vi "AprilTagFieldLayout_New.vi"(9 "FieldWidth_Meters":dbl, 10 "FieldLength_Meters":dbl, 11 "AprilTags":T1[](array[typedef]) {"POSE3D"."Translation3d"."Z" format="%14.3f"; "POSE3D"."Translation3d"."Y" format="%14.3f"; "POSE3D"."Translation3d"."X" format="%14.3f"}) -> (3 "AprilTagFieldLayout":T6={"AprilTagMap"={}, "FieldLength"=0.0, "FieldWidth"=0.0, "OriginPosition "=enum."kBlueAllianceWallRightSide,", "OriginPose3d"={"Translation3d"={"X"=0.0, "Y"=0.0, "Z"=0.0}, "Rotation3d"={"Q_quaternion"={"R"=1.0, "V"=[0.0, 0.0, 0.0]}}}} {"OriginPose3d"."Translation3d"."Z" format="%14.3f"; "OriginPose3d"."Translation3d"."Y" format="%14.3f"; "OriginPose3d"."Translation3d"."X" format="%14.3f"})   [LabVIEW 2019, in "Trajectory_Library.lvlib"]
uses:
  TypeDef/AprilTag.ctl
  TypeDef/POSE3D.ctl
  TypeDef/TRANSLATION3D.ctl
  TypeDef/ROTATION3D.ctl
  TypeDef/QUATERNION.ctl
  Trajectory_Library.lvlib
  Enum/AprilTagFieldLayoutOrignPosition_ENUM.ctl
  TypeDef/AprilTagFieldLayout.ctl
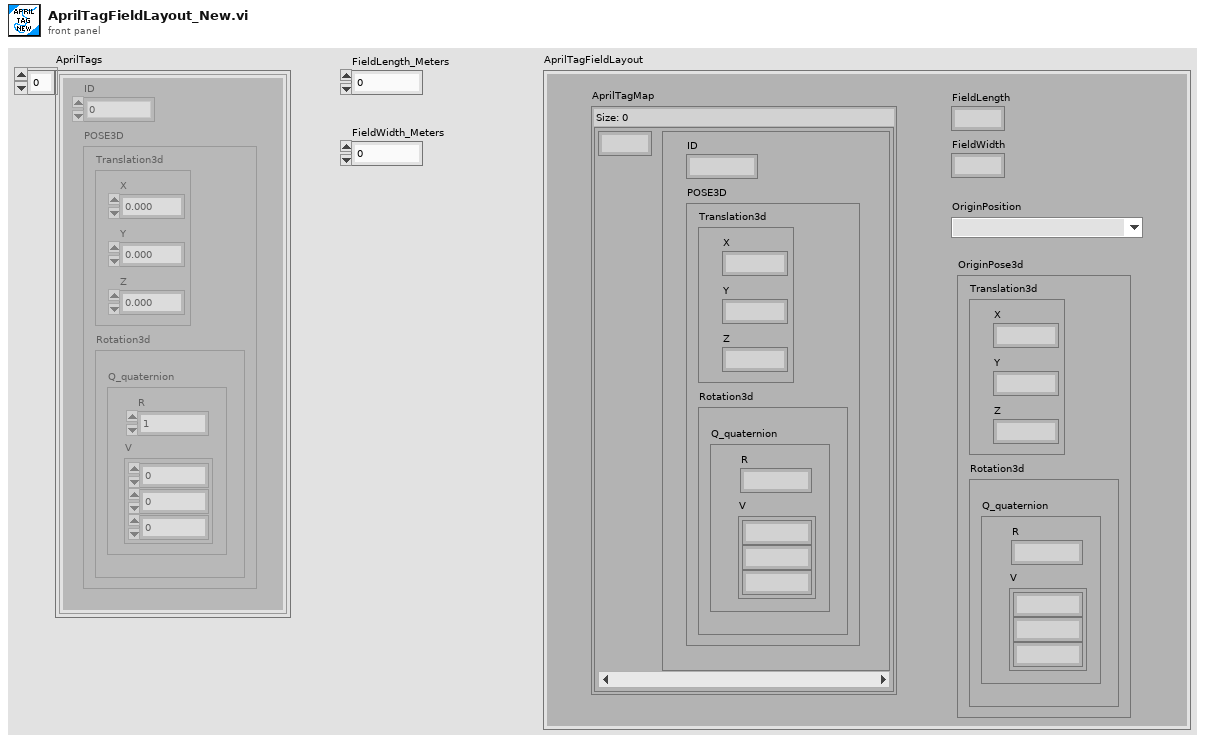
[diagram p1: front panel]
types:
  T1 = typedef "Trajectory_Library.lvlib/AprilTag.ctl" = cluster{"ID":i32, "POSE3D":T2}
  T2 = typedef "Trajectory_Library.lvlib/POSE3D.ctl" = cluster{"Translation3d":T3, "Rotation3d":T4}
  T3 = typedef "Trajectory_Library.lvlib/TRANSLATION3D.ctl" = cluster{"X":dbl, "Y":dbl, "Z":dbl}
  T4 = typedef "Trajectory_Library.lvlib/ROTATION3D.ctl" = cluster{"Q_quaternion":T5}
  T5 = typedef "Trajectory_Library.lvlib/QUATERNION.ctl" = cluster{"R":dbl, "V":dbl[]}
  T6 = typedef "Trajectory_Library.lvlib/AprilTagFieldLayout.ctl" = cluster{"AprilTagMap":map{i32, T1}, "FieldLength":dbl, "FieldWidth":dbl, "OriginPosition ":T7, "OriginPose3d":T2}
  T7 = typedef "Trajectory_Library.lvlib/AprilTagFieldLayoutOrignPosition_ENUM.ctl" = enum16{"kBlueAllianceWallRightSide,", "kRedAllianceWallRightSide,"}
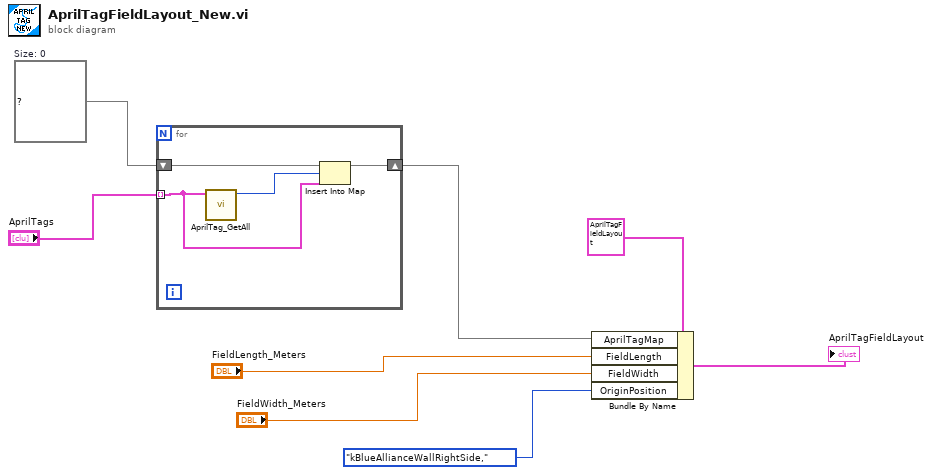
[diagram p0: block diagram]
diagram:
  w2 = map{i32, T1} {}  # Size: 0
  n1 = for {
    tunnel: "AprilTags" -> [w9] mode=indexing
    shift-right: [w12] -> w1
    shift-left: w2 -> [w11]
    n2 = call "AprilTag_GetAll.vi"("AprilTag"=w9) -> ("ID"=w10:i32)  [unwired: 9 in, 1 out]
    n3 = Insert Into Map(map in=w11, key=w10, value=w9) -> (map out=w12:map{i32, T1})  [unwired: 2 out]
  }
  n4 = Bundle By Name(cluster=T6 {"AprilTagMap"={}, "FieldLength"=0.0, "FieldWidth"=0.0, "OriginPosition "=enum."kBlueAllianceWallRightSide,", "OriginPose3d"={"Translation3d"={"X"=0.0, "Y"=0.0, "Z"=0.0}, "Rotation3d"={"Q_quaternion"={"R"=1.0, "V"=[0.0, 0.0, 0.0]}}}} ("AprilTagFieldLayout"), "AprilTagMap"=w1, "FieldLength"="FieldLength_Meters", "FieldWidth"="FieldWidth_Meters", "OriginPosition"=AprilTagFieldLayoutOrignPosition_ENUM."kBlueAllianceWallRightSide,") -> (→"AprilTagFieldLayout":T6)
